vi "array statistics.vi"(11 "Array in":dbl[](array[numeric])) -> (2 "Statistics (ms)":T1={"size "=0, "mean"=nan, "median"=nan, "min"=nan, "max"=nan} {"min" format="%#.1f"; "max" format="%#.1f"; "median" format="%.1f"; "mean" format="%.1f"})   [LabVIEW 2018, in "LV-0mq-Julia_roundtrip-lib.lvlib" / "LV2Julia_examples.lvlib"]
uses:
  LV2Julia_examples.lvlib
  statistics.ctl
  <vilib>/Analysis/baseanly.llb/Mean (DBL).vi
  <vilib>/Analysis/NI_AALBase.lvlib
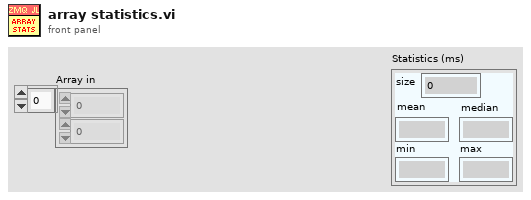
[diagram p1: front panel]
types:
  T1 = typedef "LV-0mq-Julia_roundtrip-lib.lvlib/LV2Julia_examples.lvlib/statistics.ctl" = cluster{"size ":u32, "mean":dbl, "median":dbl, "min":dbl, "max":dbl}
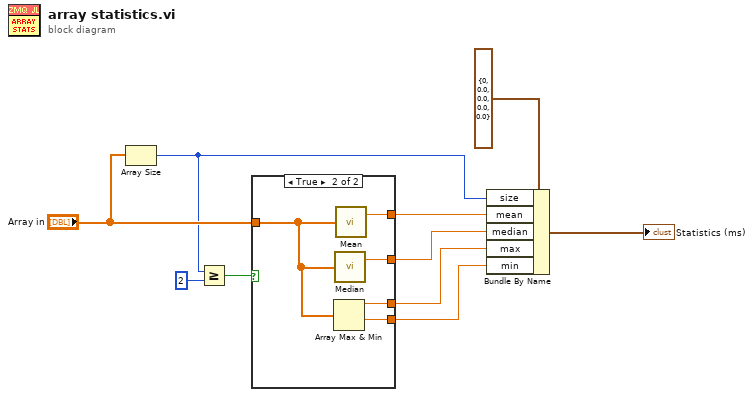
[diagram p0: block diagram]
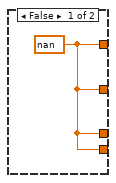
[diagram p2: hidden frame]
diagram:
  n1 = Array Size(array="Array in") -> (size(s)=w1:i32)
  n2 = Greater Or Equal?(x=w1, y=2) -> (x >= y?=w8:bool)
  n3 = case shown="True" w8 {
    tunnel: [w11 w16] -> w2
    tunnel: [w11 w15] -> w3
    tunnel: [w11 w14] -> w4
    tunnel: [w11 w13] -> w5
    tunnel: "Array in" -> [_ w12]
    frame False {
      w11 = nan ("mean")
    }
    frame True {
      n4 = Array Max & Min(array=w12) -> (max value=w15:dbl, min value=w16:dbl)  [unwired: 2 out]
      n5 = call <vilib>:"Median.vi"("X"=w12) -> ("median"=w14:dbl)  [unwired: 1 out]
      n6 = call-poly <vilib>:"Mean.vi"("X"=w12) -> ("mean"=w13:dbl)  [unwired: 1 out]
    }
  }
  n7 = Bundle By Name(cluster=T1 {"size "=0, "mean"=0.0, "median"=0.0, "min"=0.0, "max"=0.0} ("Statistics (ms)"), "size"=w1, "mean"=w5, "median"=w4, "max"=w3, "min"=w2) -> (→"Statistics (ms)":T1)
